vi "Write Metadata.vi"(8 "error in (no error)":errorcluster, 10 "Plugin Info":T2, 11 "metadata ref in":T1) -> (0 "error out":errorcluster, 3 "metadata ref dup":T1)   [LabVIEW 2021, in "CIFPluginManager.lvclass"]
uses:
  CIFPluginManager.lvclass
  <vilib>/Utility/config.llb/Config Data RefNum.ctl
  typedef/Discovered Plugin.ctl
  CIFCore/Common/Typedef/Version.ctl
  typedef/Plugin Metadata.ctl
  typedef/Loader Type.ctl
  <vilib>/Utility/config.llb/Write Key (String).vi
  <vilib>/Utility/config.llb/NI_LVConfig.lvlib
  CIFCore/Common/CIFCoreCommon.lvlib
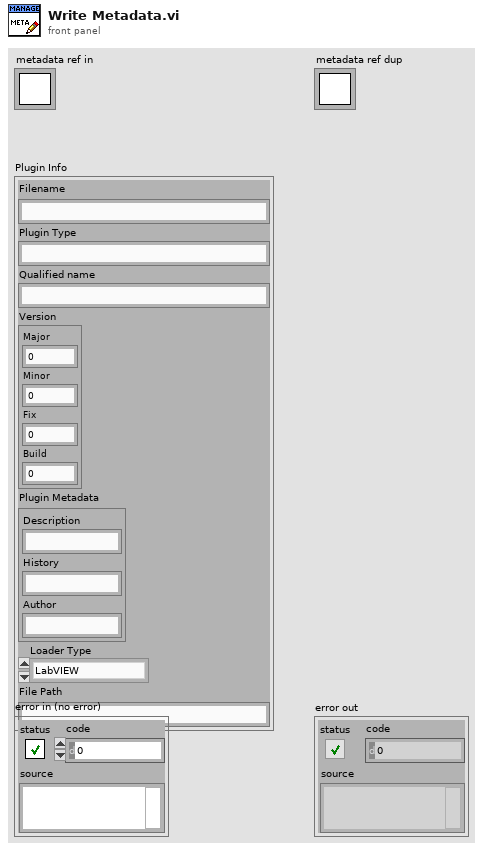
[diagram p1: front panel]
types:
  T1 = typedef "NI_LVConfig.lvlib/Config Data RefNum.ctl" = refnum<k1>
  T2 = typedef "CIFPluginManager.lvclass/Discovered Plugin.ctl" = cluster{"Filename":string, "Plugin Type":string, "Qualified name":string, "Version":T3, "Plugin Metadata":T4, "Loader Type":T5, "File Path":string}
  T3 = typedef "CIFCoreCommon.lvlib/Version.ctl" = cluster{"Major":i32, "Minor":i32, "Fix":i32, "Build":i32}
  T4 = typedef "CIFPluginManager.lvclass/Plugin Metadata.ctl" = cluster{"Description":string, "History":string, "Author":string}
  T5 = typedef "CIFPluginManager.lvclass/Loader Type.ctl" = enum16{"LabVIEW"}
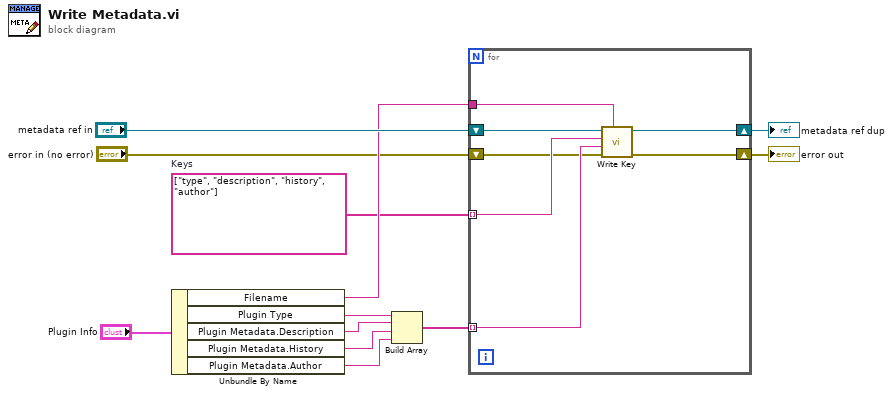
[diagram p0: block diagram]
diagram:
  w4 = string[] ["type", "description", "history", "author"]  # Keys
  n1 = Unbundle By Name("Plugin Info") -> ("Filename"=w10:string, "Plugin Type"=w9:string, "Plugin Metadata.Description"=w8:string, "Plugin Metadata.History"=w7:string, "Plugin Metadata.Author"=w6:string)
  n2 = Build Array(w9, w8, w7, w6) -> (w5:string[])
  n3 = for {
    tunnel: w10 -> [w18]
    tunnel: w5 -> [w17] mode=indexing
    tunnel: w4 -> [w16] mode=indexing
    shift-right: [w14] -> w1
    shift-left: "error in (no error)" -> [w15]
    shift-right: [w13] -> w2
    shift-left: "metadata ref in" -> [w19]
    n4 = call-poly <vilib>:"Write Key.vi"("section"=w18, "error in (no error)"=w15, "value"=w17, "key"=w16, "refnum"=w19) -> ("error out"=w14:errorcluster, "refnum out"=w13:T1)  [unwired: 4 in, 1 out]
  }
  "metadata ref dup" <- w2
  "error out" <- w1
